vi "Phasor Find Intersections of Fitted Line with Universal Circle.vi"(8 "Error In":errorcluster, 10 "Complex Coordinates":cluster{"g Array":sgl[], "s Array":sgl[]}, 11 "Phasor Array":T1[](array[typedef]) {"s" format="%#_4g"; "g" format="%#_4g"}) -> (0 "Error Out":errorcluster, 2 "Intersection 2":T1, 3 "Intersection 1":T1)   [LabVIEW 2021, in "Phasor.lvlib"]
uses:
  Phasor.lvlib
  Phasor (g, s).ctl
  <vilib>/Analysis/6fits.llb/Curve Fitting Criteria.ctl
  <vilib>/Utility/error.llb/DialogType.ctl
  4e68fa5c-e189-4374-8c1f-d16364aecb68.vi
  Utilities/Logical Processors Used.vi
  <vilib>/Utility/error.llb/Error Cluster From Error Code.vi
  <vilib>/ErrorRing/Error Ring.xnode
  <vilib>/Analysis/NI_AALPro.lvlib
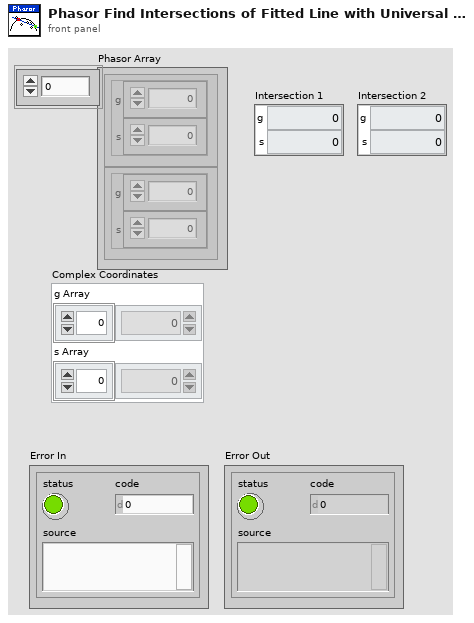
[diagram p1: front panel]
types:
  T1 = typedef "Phasor.lvlib/Phasor (g, s).ctl" = cluster{"g":dbl, "s":dbl}
  T2 = typedef "DialogType.ctl" = u16
  T3 = typedef "NI_AALPro.lvlib/Curve Fitting Criteria.ctl" = u16
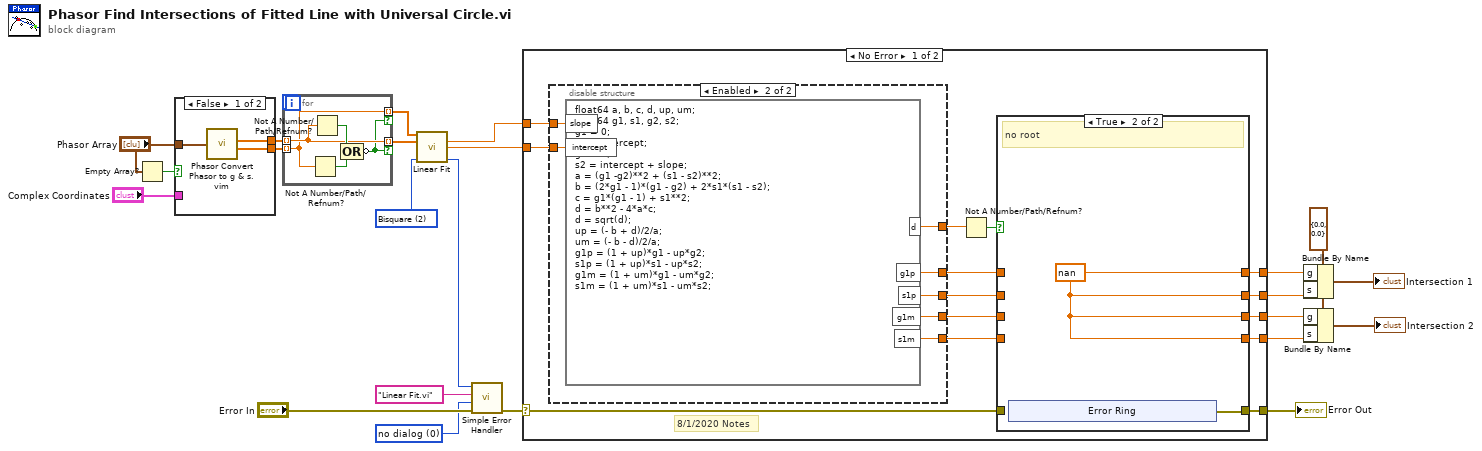
[diagram p0: block diagram]
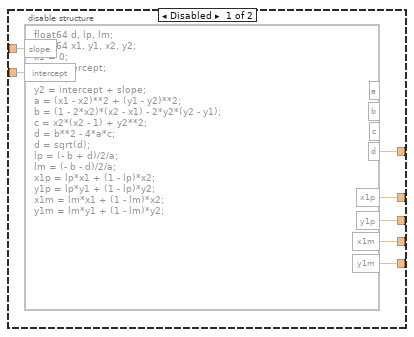
[diagram p2: hidden frame]
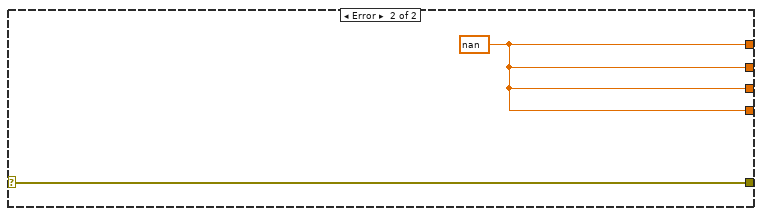
[diagram p4: hidden frame]
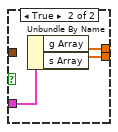
[diagram p5: hidden frame]
diagram:
  w1 = T1 {"g"=0.0, "s"=0.0} ("Intersection 1")
  w4 = T2 0 items=["no dialog", "OK message", "continue or stop message", "OK message + warnings", "continue/stop + warnings"] ("type of dialog (OK msg:1)")
  w9 = T3 2 items=["Least Square", "Least Absolute Residual", "Bisquare"] ("method")
  n1 = Empty Array?(array="Phasor Array") -> (empty?=w12:bool)
  n2 = case shown="False" w12 {
    tunnel: [w25 w28] -> w16
    tunnel: [w24 w27] -> w15
    tunnel: "Phasor Array" -> [w26 _]
    tunnel: "Complex Coordinates" -> [_ w29]
    frame False {
      n3 = call "Phasor Convert Phasor to g & s.vim"("Phasor Array"=w26) -> ("g"=w25:dbl[], "s"=w24:dbl[])  [unwired: 8 in]
    }
    frame True {
      n4 = Unbundle By Name(w29) -> ("g Array"=w28:sgl[], "s Array"=w27:sgl[])
    }
  }
  n5 = for {
    tunnel: w16 -> [w32] mode=indexing
    tunnel: w15 -> [w31] mode=indexing
    tunnel: [w32] -> w10 mode=indexing if=w30
    tunnel: [w31] -> w14 mode=indexing if=w30
    n6 = Not A Number/Path/Refnum?(number/path/refnum=w31) -> (NaN/Path/Refnum?=w34:bool)
    n7 = Not A Number/Path/Refnum?(number/path/refnum=w32) -> (NaN/Path/Refnum?=w33:bool)
    n8 = Compound Arithmetic op=OR(w33, w34) -> (invert w30:bool)
  }
  n9 = call <vilib>:"Linear Fit.vi"("Y"=w14, "X"=w10, "method"=w9) -> ("slope"=w8:dbl, "intercept"=w7:dbl, "error"=w6:i32)  [unwired: 8 in, 2 out]
  n10 = call <vilib>:"Simple Error Handler.vi"("error code (no error:0)"=w6, "error source (\" \")"="Linear Fit.vi" ("error source (\" \")"), "type of dialog (OK msg:1)"=w4, "error in (no error)"="Error In") -> ("error out"=w3:errorcluster)  [unwired: 1 in, 4 out]
  n11 = case shown="No Error" w3 {
    selector: w3 -> [w39 w75]
    tunnel: [w38 w74] -> w23
    tunnel: [w37 w74] -> w22
    tunnel: [w36 w74] -> w21
    tunnel: [w35 w74] -> w20
    tunnel: w8 -> [w48 _]
    tunnel: w7 -> [w47 _]
    tunnel: [w40 w75] -> w17
    frame No Error {
      # "8/1/2020 Notes"
      n12 = disable-structure shown="Enabled" {
        disable-tunnel: w48 -> [w55 w62]
        disable-tunnel: w47 -> [w54 w61]
        disable-tunnel: [w53 w60] -> w46
        disable-tunnel: [w52 w59] -> w44
        disable-tunnel: [w51 w58] -> w43
        disable-tunnel: [w50 w57] -> w42
        disable-tunnel: [w49 w56] -> w41
        frame Disabled {
          n13 = formula code="float64 d, lp, lm;\nfloat64 x1, y1, x2, y2;\nx1 = 0;\ny1 = intercept;\nx2 = 1;\ny2 = intercept + slope;\na = (x1 - x2)**2 + (y1 - y2)**2;\nb = (1 - 2*x2)*(x2 - x1) - 2*y2*(y2 - y1);\nc = x2*(x2 - 1) + y2**2;\nd = b**2 - 4*a*c;\nd = sqrt(d);\nlp = (- b + d)/2/a;\nlm = (- b - d)/2/a;\nx1p = lp*x1 + (1 - lp)*x2;\ny1p = lp*y1 + (1 - lp)*y2;\nx1m = lm*x1 + (1 - lm)*x2;\ny1m = lm*y1 + (1 - lm)*y2;"("slope"=w55, "intercept"=w54) -> ("x1p"=w52:dbl, "x1m"=w50:dbl, "y1p"=w51:dbl, "y1m"=w49:dbl, "d"=w53:dbl)  [unwired: 3 out]
        }
        frame Enabled {
          n14 = formula code="float64 a, b, c, d, up, um;\nfloat64 g1, s1, g2, s2;\ng1 = 0;\ns1 = intercept;\ng2 = 1;\ns2 = intercept + slope;\na = (g1 -g2)**2 + (s1 - s2)**2;\nb = (2*g1 - 1)*(g1 - g2) + 2*s1*(s1 - s2);\nc = g1*(g1 - 1) + s1**2;\nd = b**2 - 4*a*c;\nd = sqrt(d);\nup = (- b + d)/2/a;\num = (- b - d)/2/a;\ng1p = (1 + up)*g1 - up*g2;\ns1p = (1 + up)*s1 - up*s2;\ng1m = (1 + um)*g1 - um*g2;\ns1m = (1 + um)*s1 - um*s2;"("slope"=w62, "intercept"=w61) -> ("g1p"=w59:dbl, "g1m"=w57:dbl, "s1p"=w58:dbl, "s1m"=w56:dbl, "d"=w60:dbl)
        }
      }
      n15 = Not A Number/Path/Refnum?(number/path/refnum=w46) -> (NaN/Path/Refnum?=w45:bool)
      n16 = case shown="True" w45 {
        tunnel: w44 -> [w66 _]
        tunnel: w43 -> [w65 _]
        tunnel: w42 -> [w64 _]
        tunnel: w41 -> [w63 _]
        tunnel: [w67 w69] -> w40
        tunnel: w39 -> [w67 _]
        tunnel: [w66 w68] -> w38
        tunnel: [w65 w68] -> w37
        tunnel: [w64 w68] -> w36
        tunnel: [w63 w68] -> w35
        frame False {
        }
        frame True {
          w68 = sgl nan ("x1p")
          # "no root"
          n17 = xnode "Error Ring"() -> ("error out"=w69:errorcluster)
        }
      }
    }
    frame Error {
      w74 = nan ("x1p")
    }
  }
  "Error Out" <- w17
  n18 = Bundle By Name(cluster=w1, "g"=w23, "s"=w22) -> (→"Intersection 1":T1)
  n19 = Bundle By Name(cluster=w1, "g"=w21, "s"=w20) -> (→"Intersection 2":T1)
